vi "main-framework.vi"() -> ()   [LabVIEW 2017]
doc: "This template is for the Queued Message Handler design pattern.\n\nThe Event Handling Loop generates messages based on user interface actions.\n\nThe Message Handling Loop processes messages generated by the Event Handling Loop, or by other messages. The messages are string values, so new messages can be added easily to the Message Cases case structure in the Message Handling Loop. Each message cluster can also provide an optional value for Message Data, which is a variant that can be converted to whatever message-specific data is required."
uses:
  support/lib/event-message-data.ctl
  controls/UI Data.ctl
  support/Message Queue/Message Cluster.ctl
  support/Message Queue/Enqueue Message (Single).vi
  <vilib>/Utility/error.llb/Error Cluster From Error Code.vi
  <vilib>/ErrorRing/Error Ring.xnode
  support/Message Queue/Message Queue.lvlib
  support/User Event - Stop/User Event - Stop.lvlib
panel:
  out "Message":string
  out "# elements in queue":i32
  out "output cluster":T1
  in  "initial preset":T1={"command-stack"=["label1:WAIT_SECONDS,2", "LIBX,demo-testflow.vi,WAIT", "JUMPCNT,label1,1", "FINISH"], "stack-config"=""}
  out "Event Loop iteration":i32
  out "delta seconds":dbl format="%#.1g"
  out "Display <Replace Me>":string
  in  "Do Something Else <Replace Me>":bool
  in  "_PROCESS_":bool
  in  "Exit":bool
  # "r"
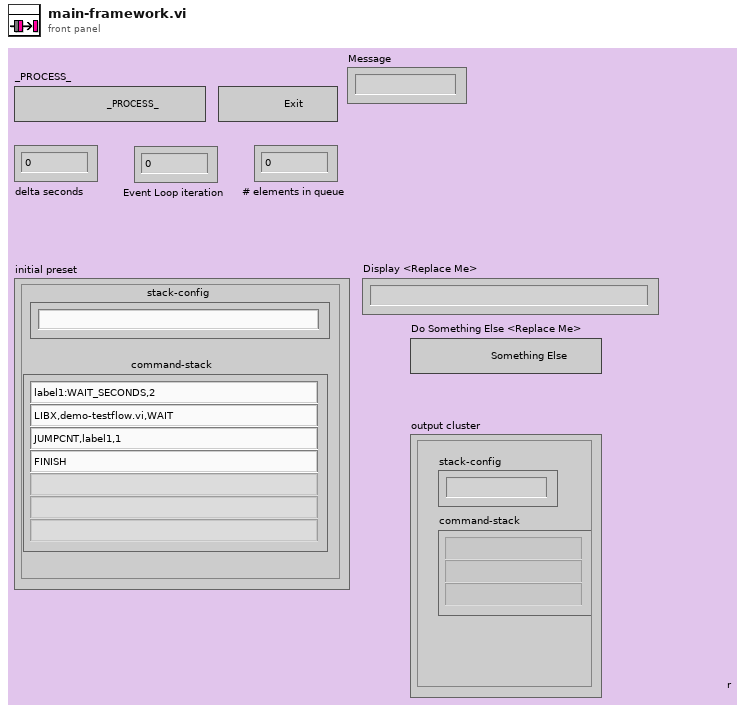
[diagram p1: front panel]
types:
  T1 = typedef "event-message-data.ctl" = cluster{"command-stack":string[], "stack-config":string}
  T2 = typedef "Message Queue.lvlib/Message Cluster.ctl" = cluster{"Message":string, "Message Data":variant}
  T3 = typedef "UI Data.ctl" = cluster{"Boolean <Replace Me>":bool, "String <Replace Me>":string, "Numeric <Replace Me>":dbl, "Do Something Ref":refnum<vi>, "Do Something Else Ref":refnum<vi>, "Data Display Ref":refnum<vi>, "Exit Button Ref":refnum<vi>}
  T4 = typedef "Message Queue.lvlib/All Message Queues.ctl" = cluster{"UI":refnum<queue>}
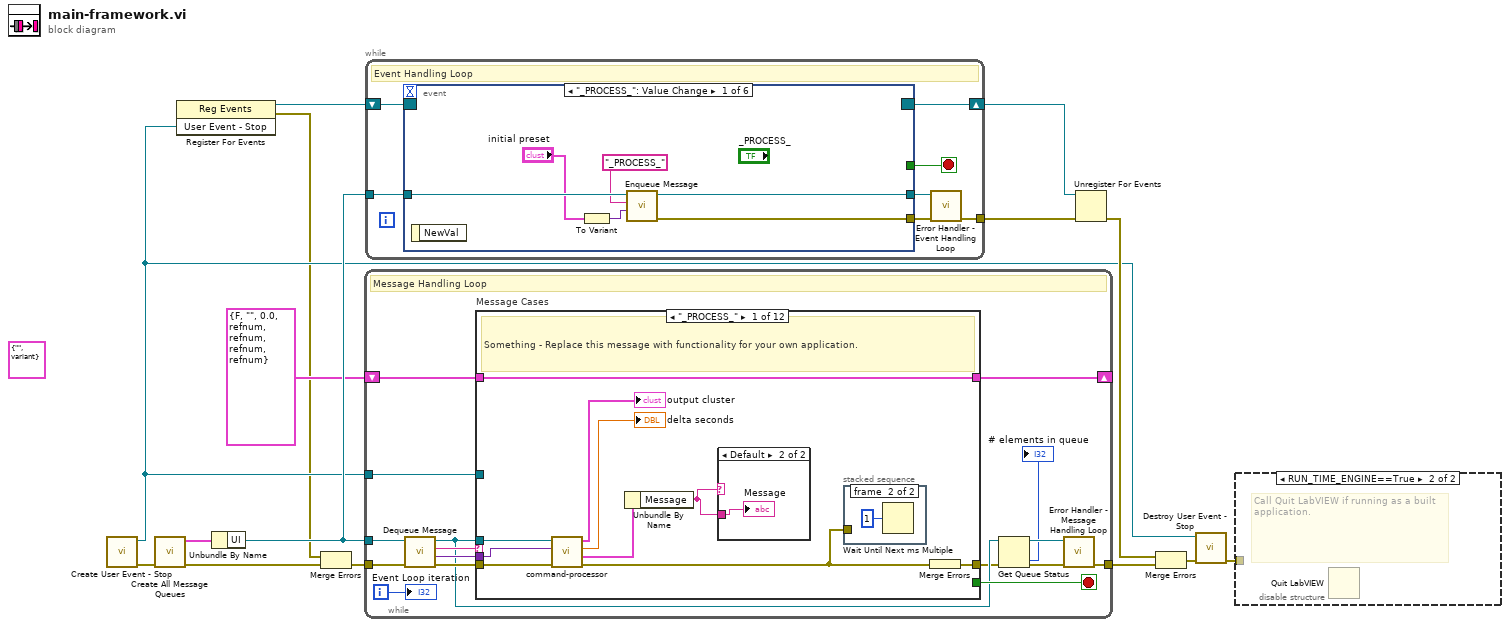
[diagram p0: block diagram]
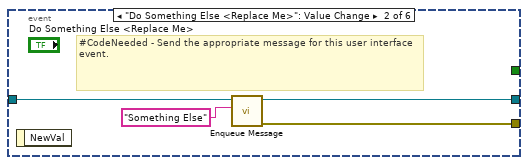
[diagram p3: hidden frame]
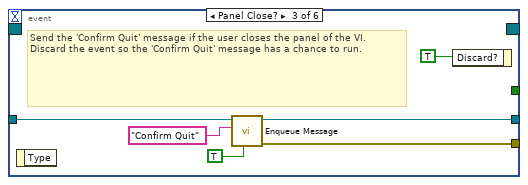
[diagram p4: hidden frame]
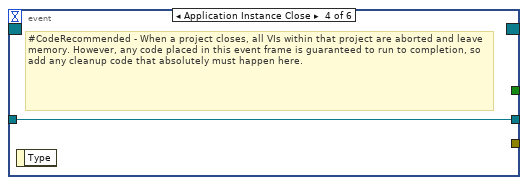
[diagram p5: hidden frame]
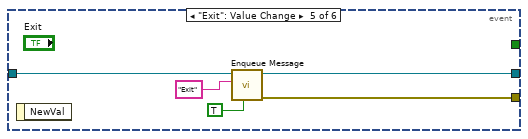
[diagram p6: hidden frame]
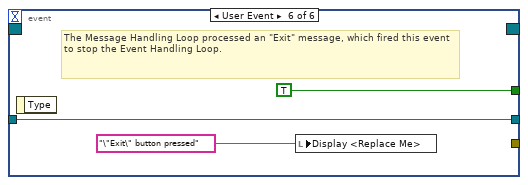
[diagram p7: hidden frame]
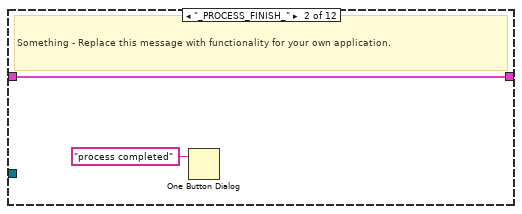
[diagram p10: hidden frame]
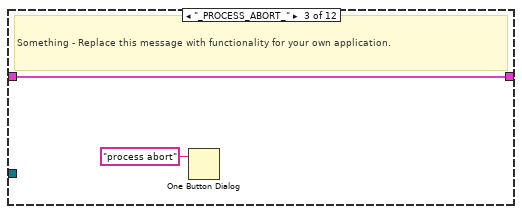
[diagram p11: hidden frame]
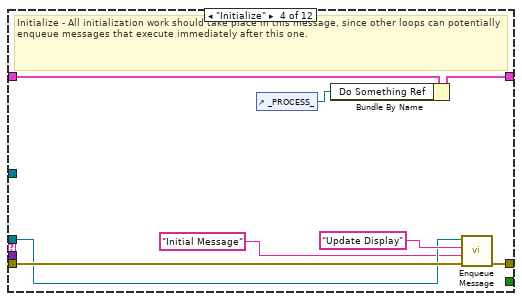
[diagram p12: hidden frame]
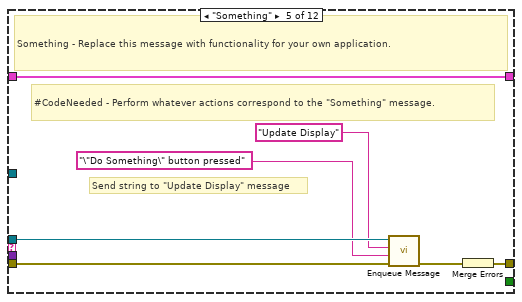
[diagram p13: hidden frame]
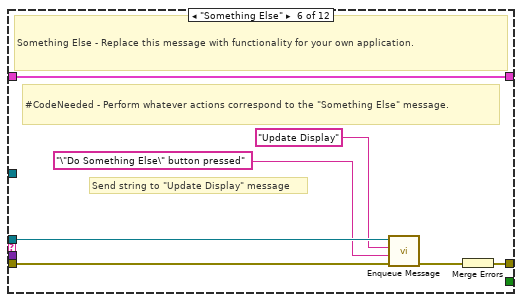
[diagram p14: hidden frame]
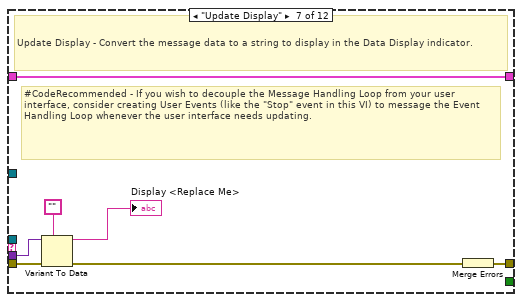
[diagram p15: hidden frame]
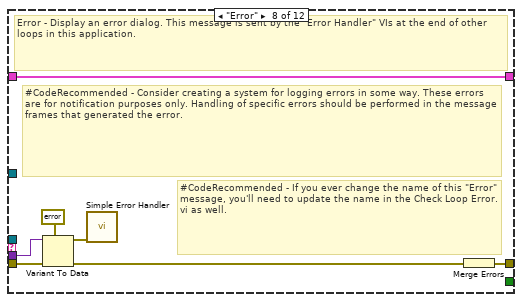
[diagram p16: hidden frame]
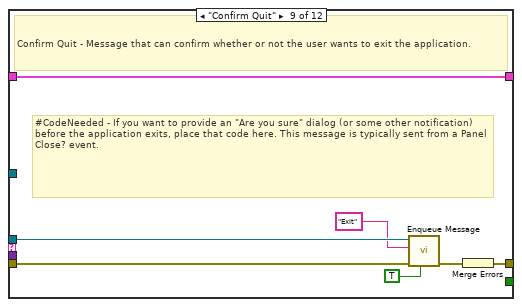
[diagram p17: hidden frame]
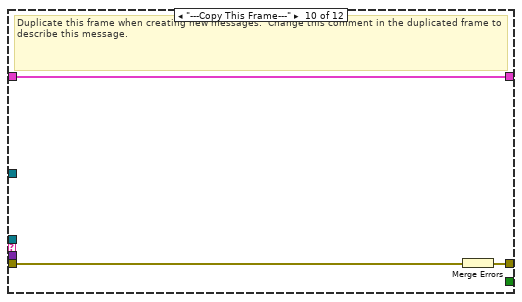
[diagram p18: hidden frame]
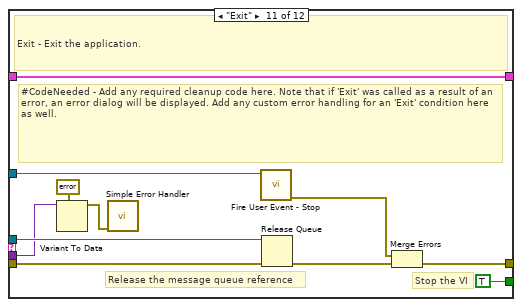
[diagram p19: hidden frame]
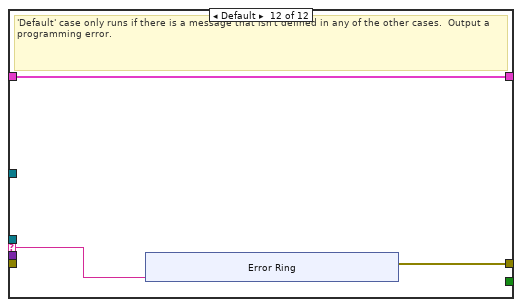
[diagram p20: hidden frame]
diagram:
  (unwired) T2 {"Message"="", "Message Data"=variant} ("Message Cluster")
  n1 = call "Create User Event - Stop.vi"() -> ("error out"=w11:errorcluster, "User Event - Stop"=w3:refnum<user-event>)  [unwired: 10 in]
  n2 = call "Create All Message Queues.vi"("error in (no error)"=w11) -> ("error out"=w15:errorcluster, "Message Queues out"=w14:T4)  [unwired: 9 in]
  n3 = register-events(w3) -> (reference out=w4:refnum<event-registration>, error out=w1:errorcluster)  [unwired: 2 in]
  n4 = Unbundle By Name(w14) -> ("UI"=w12:refnum<queue>)
  n5 = Merge Errors(w1, w15) -> (w2:errorcluster)
  n6 = while {
    tunnel: w12 -> [w23]
    shift-right: [w30] -> _
    shift-left: T3 {"Boolean <Replace Me>"=FALSE, "String <Replace Me>"="", "Numeric <Replace Me>"=0.0, "Do Something Ref"=refnum, "Do Something Else Ref"=refnum, "Data Display Ref"=refnum, "Exit Button Ref"=refnum} ("Data Cluster") -> [w31]
    tunnel: w3 -> [w28]
    tunnel: w2 -> [w27]
    tunnel: [w22] -> w13
    i -> [w21]
    stop <- w29 stop-if-true
    # "Message Handling Loop"
    n7 = call "Dequeue Message.vi"("error in (no error)"=w27, "Message Queue"=w23) -> ("error out"=w26:errorcluster, "Message Data"=w24:variant, "Message"=w25:string, "dup Message Queue"=w20:refnum<queue>)  [unwired: 6 in]
    n8 = case "Message Cases" shown="\"_PROCESS_\"" w25 {
      selector: w25 -> [_ _ _ _ _ _ _ _ _ _ _ w105]
      tunnel: w20 -> [w38 _ _ w50 w58 w65 _ _ w86 _ w104 _]
      tunnel: w26 -> [w39 _ _ w54 w60 w67 w74 w83 w90 w93 w97 _]
      tunnel: [w40 _ _ w55 w61 w68 w75 w77 w88 w91 w100 w106] -> w19
      tunnel: w31 -> [w41 w45 w47 w53 w62 w69 w76 w82 w89 w92 w103 w107]
      tunnel: [w41 w45 w47 w52 w62 w69 w76 w82 w89 w92 w103 w107] -> w30
      tunnel: [_ _ _ _ _ _ _ _ _ _ TRUE _] -> w29
      tunnel: w24 -> [w37 _ _ _ _ _ w73 w81 _ _ w94 _]
      tunnel: w28 -> [_ _ _ _ _ _ _ _ _ _ w99 _]
      frame "_PROCESS_" {
        # "Something - Replace this message with functionality for your own application."
        n9 = call "command-processor.vi"("error in"=w39, "Variant"=w37, "Queue in"=w38) -> ("error out"=w35:errorcluster, "Message Cluster 2"=w33:T2, "delta 5"=→"delta seconds":dbl, "output cluster"=→"output cluster":T1)  [unwired: 5 in]
        n10 = Unbundle By Name(w33) -> ("Message"=w32:string)
        n11 = case shown="Default" w32 {
          tunnel: w32 -> [_ w42]
          frame "\u0000" {
          }
          frame Default {
            "Message" <- w42
          }
        }
        n12 = stacked-sequence {
          tunnel: w35 -> [_ _]
          frame #0 {
          }
          frame #1 {
            n13 = Wait Until Next ms Multiple(millisecond multiple=u32 1) -> ()  [unwired: 1 out]
          }
        }
        n14 = Merge Errors(w35) -> (w40:errorcluster)
      }
      frame "_PROCESS_FINISH_" {
        # "Something - Replace this message with functionality for your own application."
        n15 = One Button Dialog(message="process completed") -> ()  [unwired: 1 in, 1 out]
      }
      frame "_PROCESS_ABORT_" {
        # "Something - Replace this message with functionality for your own application."
        n16 = One Button Dialog(message="process abort") -> ()  [unwired: 1 in, 1 out]
      }
      frame "Initialize" {
        # "Initialize - All initialization work should take place in this message, since other loops can potentially enqueue messages that execute immediately after this one."
        n17 = control-ref of="_PROCESS_"() -> (w48:refnum<vi>)
        n18 = Bundle By Name(cluster=w53, "Do Something Ref"=w48) -> (w52:T3)
        n19 = call-poly "Enqueue Message.vi"("error in (no error)"=w54, "Message Data"="Initial Message" ("Initial Message"), "Message"="Update Display", "Message Queue"=w50) -> ("error out"=w55:errorcluster)  [unwired: 6 in, 1 out]
      }
      frame "Something" {
        # "Send string to \"Update Display\" message"
        # "#CodeNeeded - Perform whatever actions correspond to the \"Something\" message."
        # "Something - Replace this message with functionality for your own application."
        n20 = call-poly "Enqueue Message.vi"("error in (no error)"=w60, "Message Data"="\"Do Something\" button pressed" ("\"Do Something\" button pressed"), "Message"="Update Display", "Message Queue"=w58) -> ("error out"=w59:errorcluster)  [unwired: 6 in, 1 out]
        n21 = Merge Errors(w59) -> (w61:errorcluster)
      }
      frame "Something Else" {
        # "Send string to \"Update Display\" message"
        # "#CodeNeeded - Perform whatever actions correspond to the \"Something Else\" message."
        # "Something Else - Replace this message with functionality for your own application."
        n22 = call-poly "Enqueue Message.vi"("error in (no error)"=w67, "Message Data"="\"Do Something Else\" button pressed" ("\"Do Something Else\" button pressed"), "Message"="Update Display", "Message Queue"=w65) -> ("error out"=w66:errorcluster)  [unwired: 6 in, 1 out]
        n23 = Merge Errors(w66) -> (w68:errorcluster)
      }
      frame "Update Display" {
        # "#CodeRecommended - If you wish to decouple the Message Handling Loop from your user interface, consider creating User Events (like the \"Stop\" event in this VI) to message the Event Handling Loop whenever the user interface needs updating."
        # "Update Display - Convert the message data to a string to display in the Data Display indicator."
        n24 = Variant To Data(error in=w74, type="", Variant=w73) -> (data=→"Display <Replace Me>":string, error out=w71:errorcluster)
        n25 = Merge Errors(w71) -> (w75:errorcluster)
      }
      frame "Error" {
        # "#CodeRecommended - If you ever change the name of this \"Error\" message, you'll need to update the name in the Check Loop Error.vi as well."
        # "#CodeRecommended - Consider creating a system for logging errors in some way. These errors are for notification purposes only. Handling of specific errors should be performed in the message frames that generated the error."
        # "Error - Display an error dialog. This message is sent by the \"Error Handler\" VIs at the end of other loops in this application."
        n26 = Variant To Data(error in=w83, type=errorcluster {"status"=FALSE, "code"=0, "source"=""} ("error constant"), Variant=w81) -> (data=w79:errorcluster, error out=w78:errorcluster)
        n27 = call <vilib>:"Simple Error Handler.vi"("error in (no error)"=w79) -> ()  [unwired: 4 in, 5 out]
        n28 = Merge Errors(w78) -> (w77:errorcluster)
      }
      frame "Confirm Quit" {
        # "#CodeNeeded - If you want to provide an \"Are you sure\" dialog (or some other notification) before the application exits, place that code here. This message is typically sent from a Panel Close? event."
        # "Confirm Quit - Message that can confirm whether or not the user wants to exit the application."
        n29 = call-poly "Enqueue Message.vi"("Priority Message? (F)"=TRUE, "error in (no error)"=w90, "Message"="Exit", "Message Queue"=w86) -> ("error out"=w87:errorcluster)  [unwired: 6 in, 1 out]
        n30 = Merge Errors(w87) -> (w88:errorcluster)
      }
      frame "---Copy This Frame---" {
        # "Duplicate this frame when creating new messages.  Change this comment in the duplicated frame to describe this message."
        n31 = Merge Errors(w93) -> (w91:errorcluster)
      }
      frame "Exit" {
        # "Stop the VI"
        # "Release the message queue reference"
        # "#CodeNeeded - Add any required cleanup code here. Note that if 'Exit' was called as a result of an error, an error dialog will be displayed. Add any custom error handling for an 'Exit' condition here as well."
        # "Exit - Exit the application."
        n32 = Variant To Data(type=errorcluster {"status"=FALSE, "code"=0, "source"=""} ("error constant"), Variant=w94) -> (data=w95:errorcluster)  [unwired: 1 in, 1 out]
        n33 = call <vilib>:"Simple Error Handler.vi"("error in (no error)"=w95) -> ()  [unwired: 4 in, 5 out]
        n34 = call "Fire User Event - Stop.vi"("User Event - Stop"=w99) -> ("error out"=w98:errorcluster)  [unwired: 10 in]
        n35 = Release Queue(queue=w104, error in (no error)=w97) -> (error out=w101:errorcluster)  [unwired: 1 in, 2 out]
        n36 = Merge Errors(w98, w101) -> (w100:errorcluster)
      }
      frame Default {
        # "'Default' case only runs if there is a message that isn't defined in any of the other cases.  Output a programming error."
        n37 = xnode "Error Ring"("parameter 0"=w105) -> ("error out"=w106:errorcluster)
      }
    }
    n38 = Get Queue Status(queue=w20, error in (no error)=w19) -> (queue out=w17:refnum<queue>, error out=w18:errorcluster, # elements in queue=→"# elements in queue":i32)  [unwired: 1 in, 5 out]
    n39 = call "Error Handler - Message Handling Loop.vi"("error in (no error)"=w18, "Message Queue"=w17) -> ("dup error in"=w22:errorcluster)  [unwired: 8 in, 1 out]
    "Event Loop iteration" <- w21
  }
  n40 = while {
    tunnel: w12 -> [w121]
    shift-right: [w119] -> w8
    shift-left: w4 -> [w120]
    tunnel: [w115] -> w5
    stop <- w117 stop-if-true
    # "Event Handling Loop"
    n41 = event shown="[0] \"_PROCESS_\": Value Change" {
      selector: w120 -> [_ _ _ _ _ _]
      dyn-events: [_ _ _ _ _ _] -> w119
      timeout: _ -> [_ _ _ _ _ _]
      tunnel: [_ _ _ _ _ TRUE ("Discard?")] -> w117
      tunnel: w121 -> [w127 w131 w136 w138 w143 w146]
      tunnel: [w124 w128 w135 _ w142 _] -> w118
      tunnel: [w126 w130 w134 w138 w141 w146] -> w116
      event "_PROCESS_": Value Change {
        n42 = event-data() -> ()  [unwired: 1 in, 1 out]
        n43 = To Variant(anything="initial preset") -> (Variant=w122:variant)
        n44 = call-poly "Enqueue Message.vi"("Message Data"=w122, "Message"="_PROCESS_", "Message Queue"=w127) -> ("error out"=w124:errorcluster, "dup Message Queue"=w126:refnum<queue>)  [unwired: 7 in]
      }
      event "Do Something Else <Replace Me>": Value Change {
        # "#CodeNeeded - Send the appropriate message for this user interface event."
        n45 = event-data() -> ()  [unwired: 1 in, 1 out]
        n46 = call-poly "Enqueue Message.vi"("Message"="Something Else", "Message Queue"=w131) -> ("error out"=w128:errorcluster, "dup Message Queue"=w130:refnum<queue>)  [unwired: 8 in]
      }
      event Panel Close? {
        # "Send the 'Confirm Quit' message if the user closes the panel of the VI. Discard the event so the 'Confirm Quit' message has a chance to run."
        n47 = event-data() -> ()  [unwired: 1 in, 1 out]
        n48 = call-poly "Enqueue Message.vi"("Priority Message? (F)"=TRUE, "Message"="Confirm Quit", "Message Queue"=w136) -> ("error out"=w135:errorcluster, "dup Message Queue"=w134:refnum<queue>)  [unwired: 7 in]
        n49 = event-data("Discard?"=TRUE) -> ()  [unwired: 1 in, 1 out]
      }
      event Application Instance Close {
        # "#CodeRecommended - When a project closes, all VIs within that project are aborted and leave memory. However, any code placed in this event frame is guaranteed to run to completion, so add any cleanup code that absolutely must happen here."
        n50 = event-data() -> ()  [unwired: 1 in, 1 out]
      }
      event "Exit": Value Change {
        n51 = event-data() -> ()  [unwired: 1 in, 1 out]
        n52 = call-poly "Enqueue Message.vi"("Priority Message? (F)"=TRUE, "Message"="Exit", "Message Queue"=w143) -> ("error out"=w142:errorcluster, "dup Message Queue"=w141:refnum<queue>)  [unwired: 7 in]
      }
      event User Event {
        # "The Message Handling Loop processed an \"Exit\" message, which fired this event to stop the Event Handling Loop."
        n53 = event-data() -> ()  [unwired: 1 in, 1 out]
        n54 = local write "Display <Replace Me>"("\"Exit\" button pressed" ("VI Stopped")) -> ()
      }
    }
    n55 = call "Error Handler - Event Handling Loop.vi"("error in (no error)"=w118, "Message Queue"=w116) -> ("dup error in"=w115:errorcluster)  [unwired: 8 in, 1 out]
  }
  n56 = Unregister For Events(event registration refnum=w8, error in=w5) -> (error out=w9:errorcluster)
  n57 = Merge Errors(w9, w13) -> (w10:errorcluster)
  n58 = call "Destroy User Event - Stop.vi"("error in (no error)"=w10, "User Event - Stop"=w3) -> ("error out"=w6:errorcluster)  [unwired: 9 in]
  n59 = disable-structure shown="RUN_TIME_ENGINE==True" {
    disable-tunnel: w6 -> [_ _]
    frame condition #0 (active) {
    }
    frame condition #1 {
      # "Call Quit LabVIEW if running as a built application."
      n60 = Quit LabVIEW() -> ()  [unwired: 1 in]
    }
  }
